vi "Configure Device.vi"(8 "error in (no error)":errorcluster, 11 "Simulated PSU in":refnum<class "Simulated PSU.lvclass">) -> (0 "error out":errorcluster, 3 "Simulated PSU out":refnum<class "Simulated PSU.lvclass">)   [LabVIEW 2020, in "Simulated PSU.lvlib" / "Simulated PSU.lvclass"]
uses:
  Simulated PSU.lvclass
  Simulated PSU.lvclass/Simulated PSU.ctl
  build/ppl/lv-hal.lvlibp/Device/Device.lvclass
  C:/dev/HAL Demo/build/ppl/lv-hal.lvlibp/Device/Device.lvclass
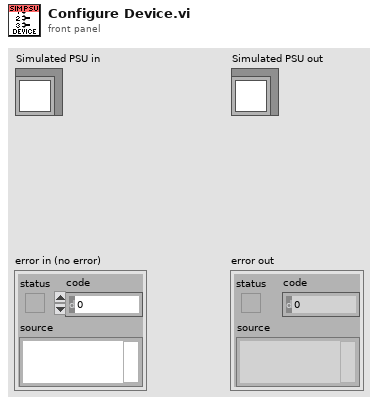
[diagram p1: front panel]
types:
  T1 = typedef "Simulated PSU.lvlib/Simulated PSU.lvclass/Ref Data.ctl" = cluster{"Enabled":bool, "Voltage":dbl, "Noise Level":dbl, "Resistance":dbl}
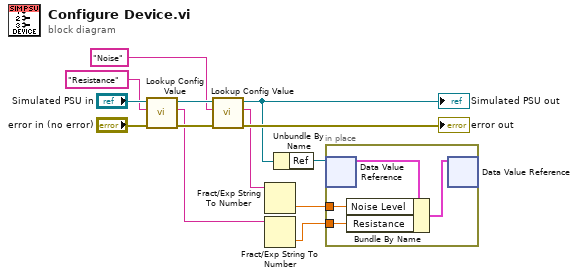
[diagram p0: block diagram]
diagram:
  n1 = call "Lookup Config Value.vi"("error in (no error)"="error in (no error)", "Config Key"="Resistance", "Device in"="Simulated PSU in") -> ("error out"=w9:errorcluster, "Value"=w6:string, "Device out"=w10:refnum<class "Simulated PSU.lvclass">)  [unwired: 5 in, 1 out]
  n2 = call "Lookup Config Value.vi"("error in (no error)"=w9, "Config Key"="Noise", "Device in"=w10) -> ("error out"=→"error out":errorcluster, "Value"=w5:string, "Device out"=w3:refnum<class "Simulated PSU.lvclass">)  [unwired: 5 in, 1 out]
  "Simulated PSU out" <- w3
  n3 = Fract/Exp String To Number(string=w5) -> (number=w2:dbl)  [unwired: 3 in, 1 out]
  n4 = Fract/Exp String To Number(string=w6) -> (number=w1:dbl)  [unwired: 3 in, 1 out]
  n5 = Unbundle By Name(w3) -> ("Ref"=w4:refnum<data-value>)
  n6 = in-place {
    in-place-border: w2 -> [w15]
    in-place-border: w1 -> [w14]
    n7 = in-place-dvr #1(w4) -> (w17:T1)  [unwired: 1 out]
    n8 = Bundle By Name(cluster=w17, "Noise Level"=w15, "Resistance"=w14) -> (w16:T1)
    n9 = in-place-dvr #1(w16) -> ()  [unwired: 2 out]
  }
